vi "Init_All_FPGAs.vi"(8 "error in (no error)":errorcluster, 11 "Array":cluster{"HWMd":T1, "Data":variant}[](array[cluster])) -> (0 "error out":errorcluster)   [LabVIEW 2018]
uses:
  Queue/HWQueueElements.ctl
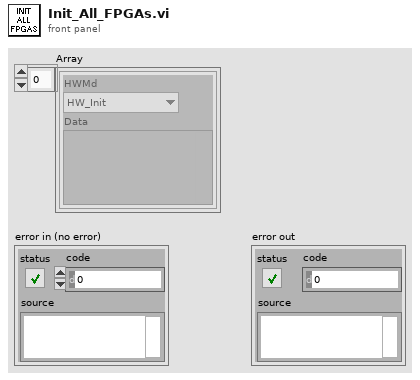
[diagram p1: front panel]
types:
  T1 = typedef "HWQueueElements.ctl" = enum16{"HW_Init", "HW_UpdtCfg", "HW_Start", "HW_Pause", "HW_Run", "HW_Cls", "HW_Exit"}
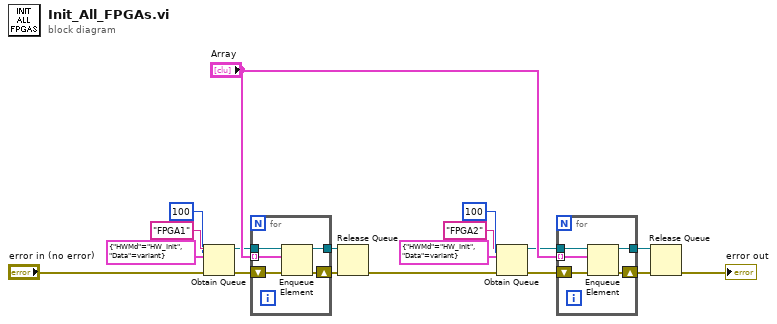
[diagram p0: block diagram]
diagram:
  n1 = Obtain Queue(max queue size (-1, unlimited)=100, name (unnamed)="FPGA1", element data type=cluster{"HWMd":T1, "Data":variant} {"HWMd"=enum."HW_Init", "Data"=variant}, error in (no error)="error in (no error)") -> (queue out=w11:refnum<queue>, error out=w10:errorcluster)  [unwired: 1 in, 1 out]
  n2 = for {
    tunnel: w11 -> [w22]
    shift-right: [w21] -> w6
    shift-left: w10 -> [w23]
    tunnel: "Array" -> [w20] mode=indexing
    tunnel: [w19] -> w4
    n3 = Enqueue Element(queue=w22, element=w20, error in (no error)=w23) -> (queue out=w19:refnum<queue>, error out=w21:errorcluster)  [unwired: 1 in, 1 out]
  }
  n4 = Release Queue(queue=w4, error in (no error)=w6) -> (error out=w5:errorcluster)  [unwired: 1 in, 2 out]
  n5 = Obtain Queue(max queue size (-1, unlimited)=100, name (unnamed)="FPGA2", element data type=cluster{"HWMd":T1, "Data":variant} {"HWMd"=enum."HW_Init", "Data"=variant}, error in (no error)=w5) -> (queue out=w12:refnum<queue>, error out=w13:errorcluster)  [unwired: 1 in, 1 out]
  n6 = for {
    tunnel: w12 -> [w27]
    shift-right: [w26] -> w3
    shift-left: w13 -> [w28]
    tunnel: "Array" -> [w25] mode=indexing
    tunnel: [w24] -> w1
    n7 = Enqueue Element(queue=w27, element=w25, error in (no error)=w28) -> (queue out=w24:refnum<queue>, error out=w26:errorcluster)  [unwired: 1 in, 1 out]
  }
  n8 = Release Queue(queue=w1, error in (no error)=w3) -> (error out=→"error out":errorcluster)  [unwired: 1 in, 2 out]
